vi "Working distances and rectangle.vi"() -> ()   [LabVIEW 2017]
uses:
  <vilib>/Simulation/Scripting/Companion Diagram/SimConfigNode/SimParams.ctl
  <vilib>/Simulation/Scripting/Companion Diagram/SimConfigNode/_simSolvers.ctl
  <vilib>/Simulation/Implementation/Shared/SIMSCR Execution Mode.ctl
  <vilib>/Simulation/Param Hierarchy/Typedefs/SIMPH Param Control Actions.ctl
  <vilib>/Simulation/Implementation/Shared/NILVSim_ParamChanged.vi
  <vilib>/Simulation/Implementation/Shared/NILVSIM_BeginStep.vi
  <vilib>/Simulation/Implementation/Shared/NILVSim_Manager.vi
  <vilib>/Utility/error.llb/Clear Errors.vi
  <vilib>/Simulation/Implementation/Shared/NILVSim_FinalizeModel.vi
  <vilib>/DAQmx/read.llb/DAQmx Read (Counter DBL 1Chan 1Samp).vi
  <vilib>/DAQmx/read.llb/DAQmx Read (Digital Bool 1Line 1Point).vi
  917b7e52-755f-4d44-bea8-9e7c9beac24e.vi
  a58f9967-76f1-4ebc-ad3d-26e75a3ca160.vi
  <vilib>/DAQmx/write.llb/DAQmx Write (Analog DBL 1Chan 1Samp).vi
  <vilib>/DAQmx/create/channels.llb/DAQmx Create Channel (AO-Voltage-Basic).vi
  <vilib>/DAQmx/create/channels.llb/DAQmx Create Channel (DI-Digital Input).vi
  <vilib>/DAQmx/create/channels.llb/DAQmx Create Channel (CI-Count Edges).vi
  <vilib>/Simulation/Implementation/Shared/SIM Unbundle Sim Info.vi
  <vilib>/Simulation/Implementation/Shared/NILVSim_Initialize.vi
  <vilib>/Simulation/Utility/Implementation/NILVSim Get Time and IsAcceptedStep.vi
  <vilib>/Simulation/Implementation/Shared/SIMSH Read Queue.vi
  <vilib>/Simulation/Implementation/Shared/NILVSim_GetModelError.vi
  <vilib>/Simulation/Implementation/Shared/SIM Bundle Sim Info.vi
  <vilib>/DAQmx/miscellaneous.llb/DAQmx Fill In Error Info.vi
  <vilib>/Simulation/Implementation/XNodeFramework/SimXNode/SimX.xnode
  <vilib>/Simulation/Model Libraries/PID/SIM PID (Parallel).vi
  <vilib>/Simulation/Model Libraries/PID/SIM PID.vi
  <vilib>/Simulation/Scripting/Companion Diagram/SimConfigNode/SimDog.xnode
  <vilib>/Simulation/Model Libraries/PID/SIM PID (Academic).vi
  <vilib>/Simulation/Implementation/Shared/NI_SIM_Implementation.lvlib
panel:
  out "circle reset":bool
  in  "part circle":enum16{"d", "c", "b", "a"}(ring)
  in  "Raduis":dbl
  out "at 2f":bool
  out "Step 2J":bool
  out "Step 2H":bool
  out "Shape drawing steps":enum16{"corner", "1st switch", "reverse"}(ring)
  out "Step 2D":bool
  out "Step 2C":bool
  out "c":bool
  in  "height":dbl
  in  "length":dbl
  in  "part":T1(ring)=enum."a"
  out "Step 2A":bool
  out "Step 2B":bool
  in  "Has encoders been reset?":enum16{"don't reset", "reset"}(ring)
  out "x distance currently being travelled":dbl
  out "y distance currently being travelled":dbl
  out "error calced":dbl
  out "p1 dis 2":dbl
  out "p1 dis":dbl
  out "error y":dbl
  out "calc distance y":dbl
  out "Boolean 2":bool
  out "calc distanc x":dbl
  out "error":dbl
  out "reached1":bool
  out "reached":bool
  out "Numeric":dbl
  in  "Draw rectangle":bool
  in  "Draw circle":bool
  out "In drawing mode":bool
  in  "Right-Down":bool
  in  "Left-Up":bool
  in  "Left-Down":bool
  in  "Right-Up":bool
  in  "right":bool
  in  "left":bool
  in  "motor 2":dbl(slide)=1.5 scale=-10.0..10.0
  in  "down":bool
  in  "up":bool
  in  "Y Length":dbl=30.0
  in  "X Length":dbl=30.0
  in  "Motor 2 encoder":tag="Dev1/ctr1"
  out "Pulses M2":dbl format="%.2f"
  in  "Motor 1 encoder":tag="Dev1/ctr0"
  out "Pulses M1":dbl format="%.2f"
  out "Right":bool
  out "Bottom":bool
  out "Left":bool
  out "Top":bool
  in  "Switch 4/Line 3":tag="Dev1/port0/line3"
  in  "Switch 3/Line 2":tag="Dev1/port0/line2"
  in  "Switch 2/Line 1":tag="Dev1/port0/line1"
  in  "Switch 1/Line 0":tag="Dev1/port0/line0"
  in  "Motor stop":bool
  in  "Motor 1":tag="Dev1/ao0"
  in  "max Voltage":dbl=10.0
  in  "Min Voltage":dbl=-10.0
  in  "Motor 2":tag="Dev1/ao1"
  in  "motor 1":dbl(slide)=1.5 scale=-10.0..10.0
  in  "stop":bool
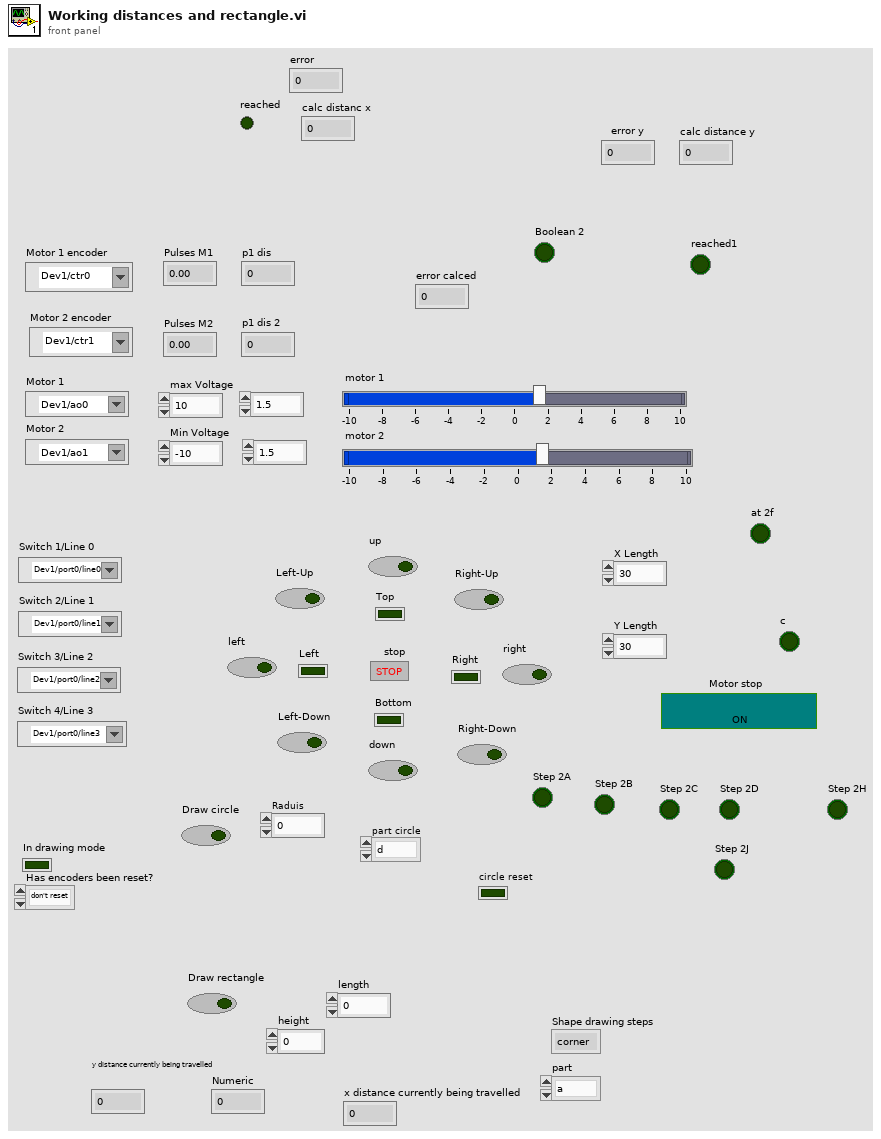
[diagram p1: front panel]
types:
  T1 = enum16{"nothing", "j", "i", "h", "g", "f", "e", "d", "c", "b", "a"}
  T2 = enum16{"Simulate to Completion", "Single Time-Step Simulation (Fixed Step Only)"}
  T3 = typedef "SIMSCR Execution Mode.ctl" = enum16{"Simulate to Completion", "Single Time-Step Simulation (Fixed Step Only)"}
  T4 = typedef "SIMPH Param Control Actions.ctl" = enum16{"get params", "set params"}
  T5 = cluster{"SIMSH Sim Time":dbl, "SIM PID Derivative Gain.vi":cluster{"output":dbl}, "SIM PID Derivative Gain.vi - SIMSH":cluster{"SIMSH Sim Time":dbl, "t 3":dbl, "Select 2":cluster{"s? t:f":dbl}, "Equal?":cluster{"x = y?":bool}, "Or":cluster{"x .or. y?":bool}, "Equal To 0?":cluster{"x = 0?":bool}}, "High Frequency [s] (Tf)":dbl, "Gain":cluster{"output":dbl}, "Summation":cluster{"Result":dbl}, "Integral Gain - series.vi":cluster{"output":dbl}, "Integral Gain - series.vi - SIMSH":cluster{"SIMSH Sim Time":dbl, "Select 2":cluster{"s? t:f":dbl}, "integral in gain?":bool, "Integrator":cluster{"output y(t)":dbl}, "Gain 2":cluster{"output":dbl}, "Select":cluster{"s? t:f":dbl}, "Equal To 0?":cluster{"x = 0?":bool}, "Reciprocal":cluster{"1/x":dbl}}}
  T6 = typedef "SimParams.ctl" = cluster{"Initial Time (s)":dbl, "Final Time (s)":dbl, "Step Size (s)":dbl, "ODE Solver":T7, "Minimum Step Size (s)":dbl, "Maximum Step Size (s)":dbl, "Relative Tolerance":dbl, "Absolute Tolerance":dbl, "Software Timing":bool, "Initial Step Size (s)":dbl, "Automatic Fixed Step Size?":bool, "Automatic Discrete Step Size?":bool, "Discrete Step Size (s)":dbl, "Calculate using Time Step":bool, "Solver Wired?":bool, "Prev.Frm.Expected End":u64, "Prev.Frm.Actual End":u64, "Prev.Frm.Finished Late?":bool, "Prev.Iter.Expected End":u64, "Prev.Iter.Actual End":u64, "Prev.Iter.Finished Late?":bool, "Expected Iteration Start":u64, "Actual Iteration Start":u64, "Expected Frame Start":u64, "Actual Frame Start":u64, "Source Name":string, "Name":string, "Period":i64, "Deadline":i64, "Offset":i64, "Start":i64, "Priority":i32, "Timeout":i32, "Processor":i32, "Mode":enum32{"No Change", "Process missed periods, maintain original phase", "Discard missed periods, maintain original phase", "Process missed periods, ignore original phase", "Discard missed periods, ignore original phase"}, "Wakeup reason":enum32{"Normal", "Aborted", "Asynchronous wakeup", "Timing source error", "Timed loop error", "Timeout"}, "Error":errorcluster, "Source Type":string, "Secondary Source Type":string, "Global End Time":u64, "Global Start Time":u64, "Full Solver Reset":bool, "Execution Mode":T3, "Nan/Inf Check":bool, "Custom Solver Library":string, "Solver Is Variable":bool, "custom solver name":string, "Signal Collection Decimation":u32}
  T7 = typedef "_simSolvers.ctl" = enum16{"Runge-Kutta 1 (Euler)", "Runge-Kutta 2", "Runge-Kutta 3", "Runge-Kutta 4", "Runge-Kutta 23 (variable)", "Runge-Kutta 45 (variable)", "BDF (variable)", "Adams-Moulton (variable)", "Rosenbrock (variable)", "Discrete States Only", "SDIRK 4 (variable)", "Radau 5 (variable)", "Radau 9 (variable)", "Radau 13 (variable)", "Radau [Variable Order] (variable)", "Gear's Method (variable)", "Linearizer", "State Query", "Trim Eval", "Custom Solver"}
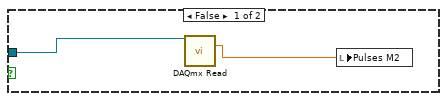
[diagram p2: hidden frame]
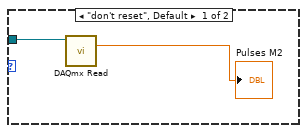
[diagram p3: hidden frame]
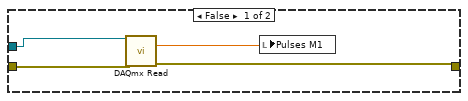
[diagram p4: hidden frame]
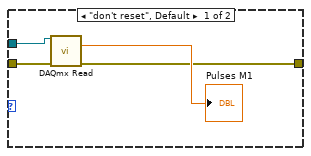
[diagram p5: hidden frame]
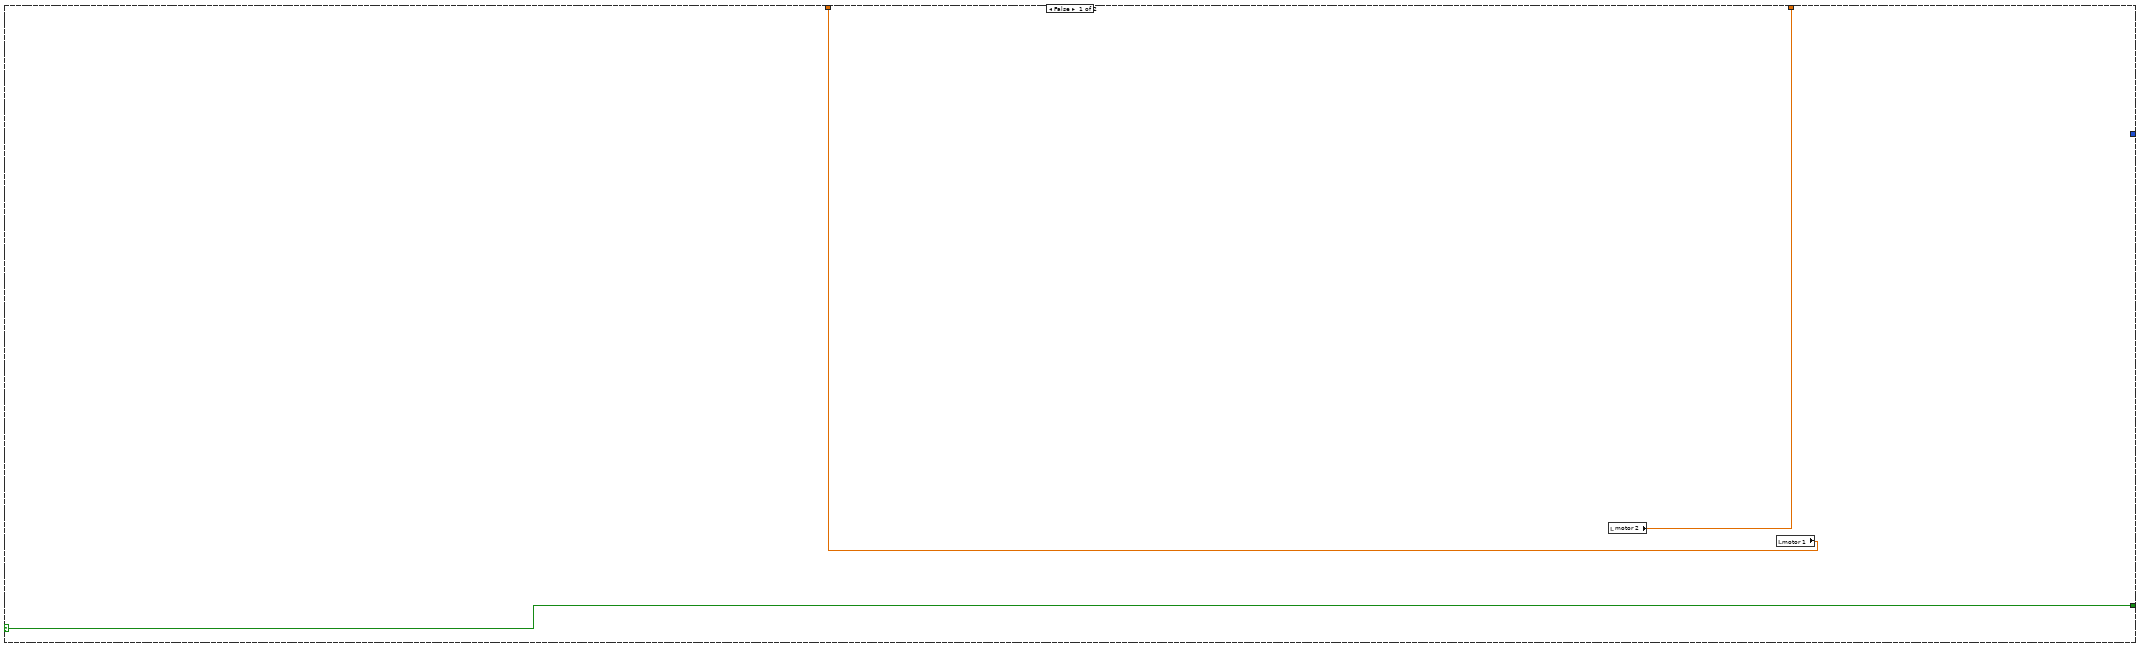
[diagram p6: hidden frame]
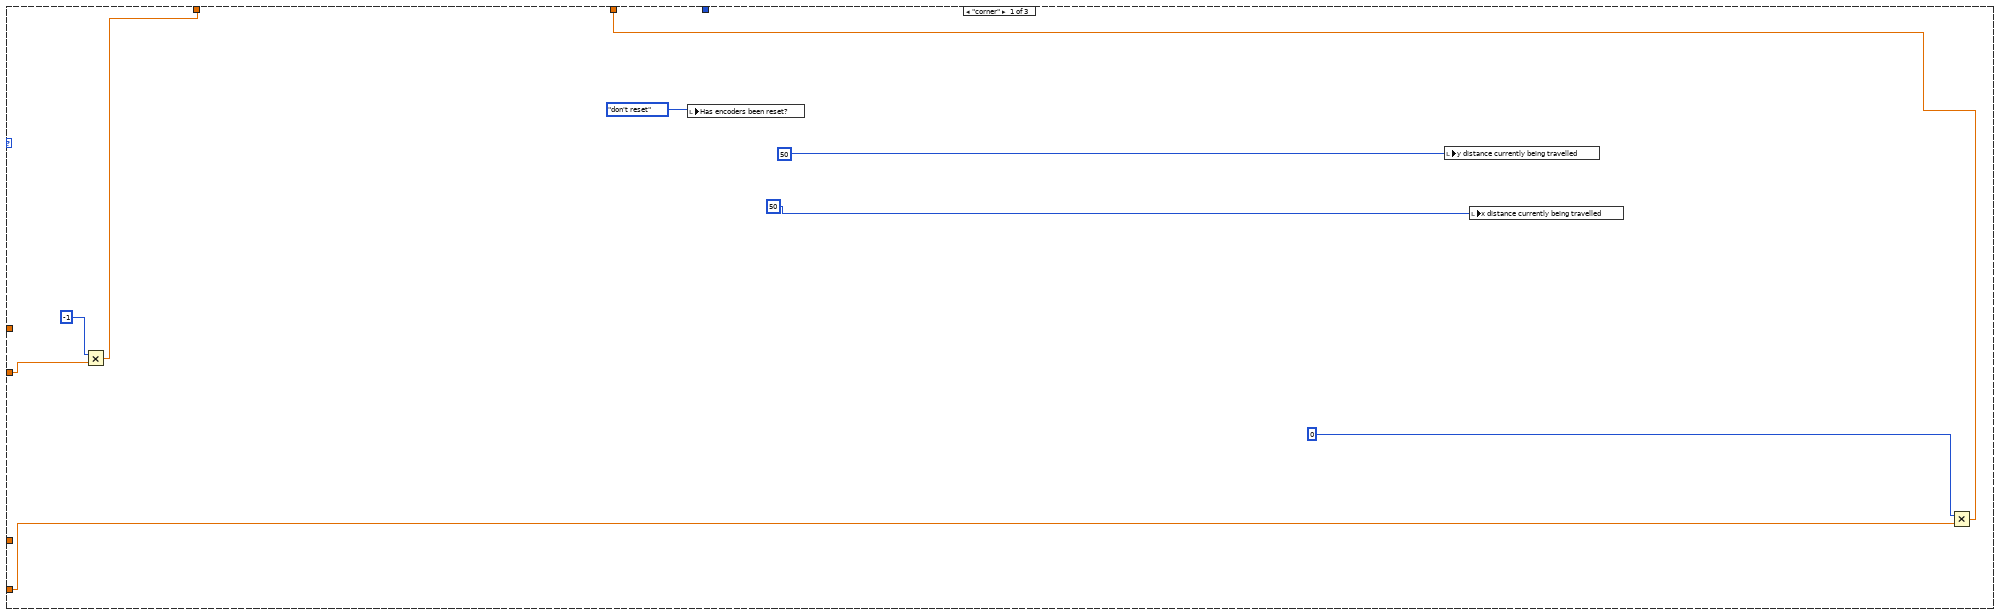
[diagram p7: hidden frame]
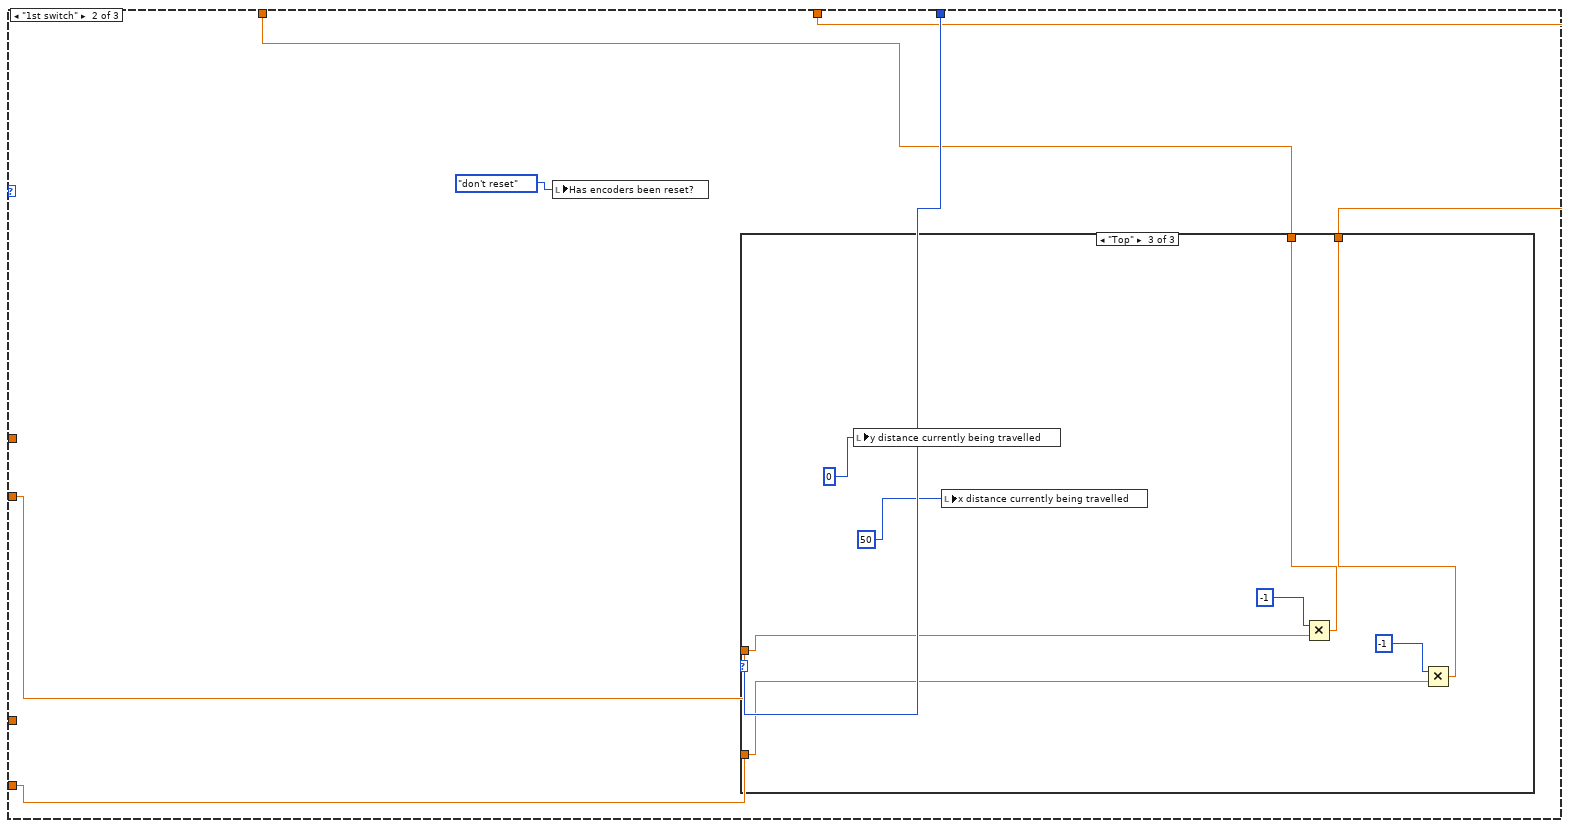
[diagram p8: hidden frame]
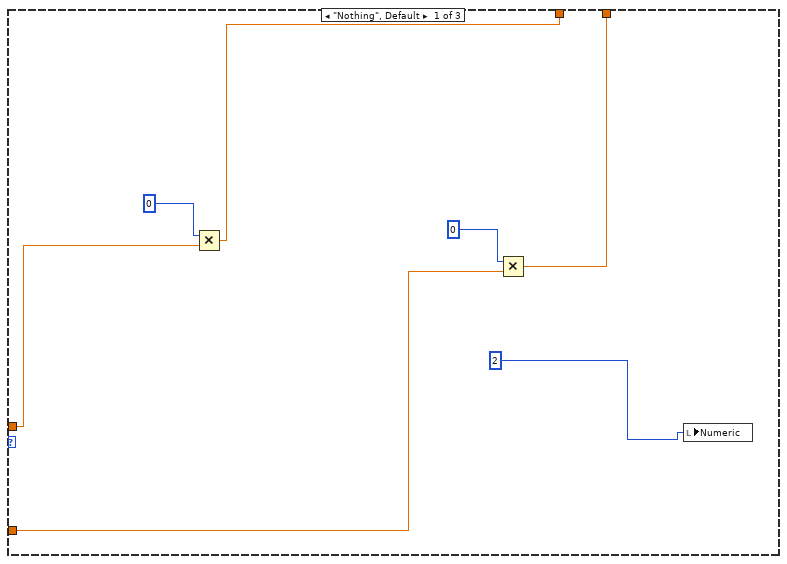
[diagram p9: hidden frame]
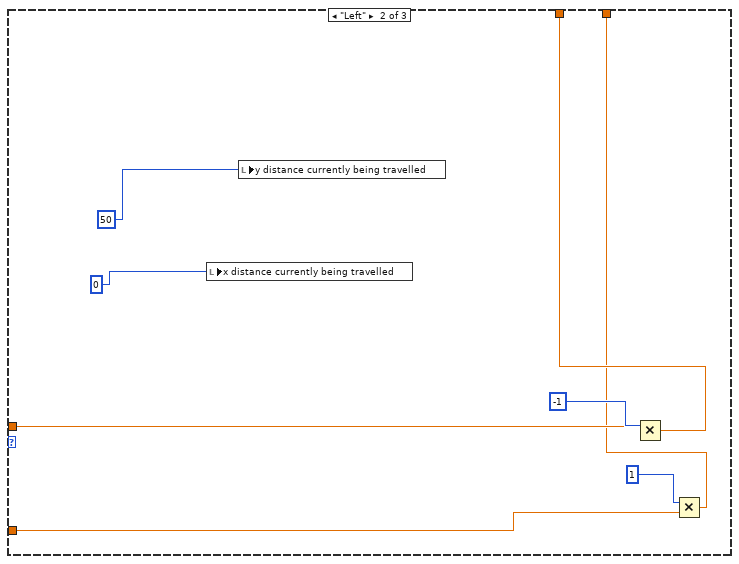
[diagram p10: hidden frame]
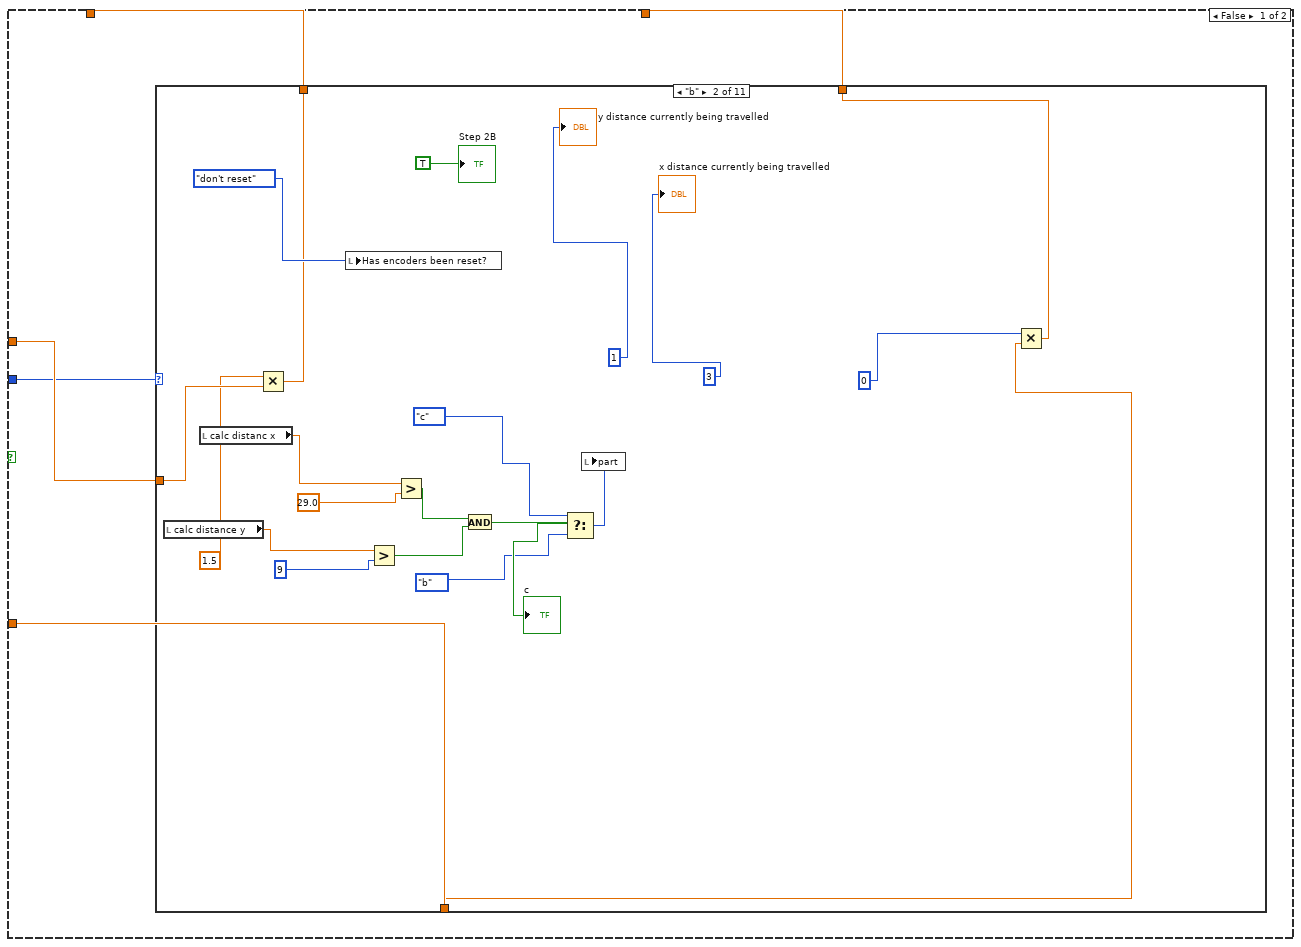
[diagram p11: hidden frame]
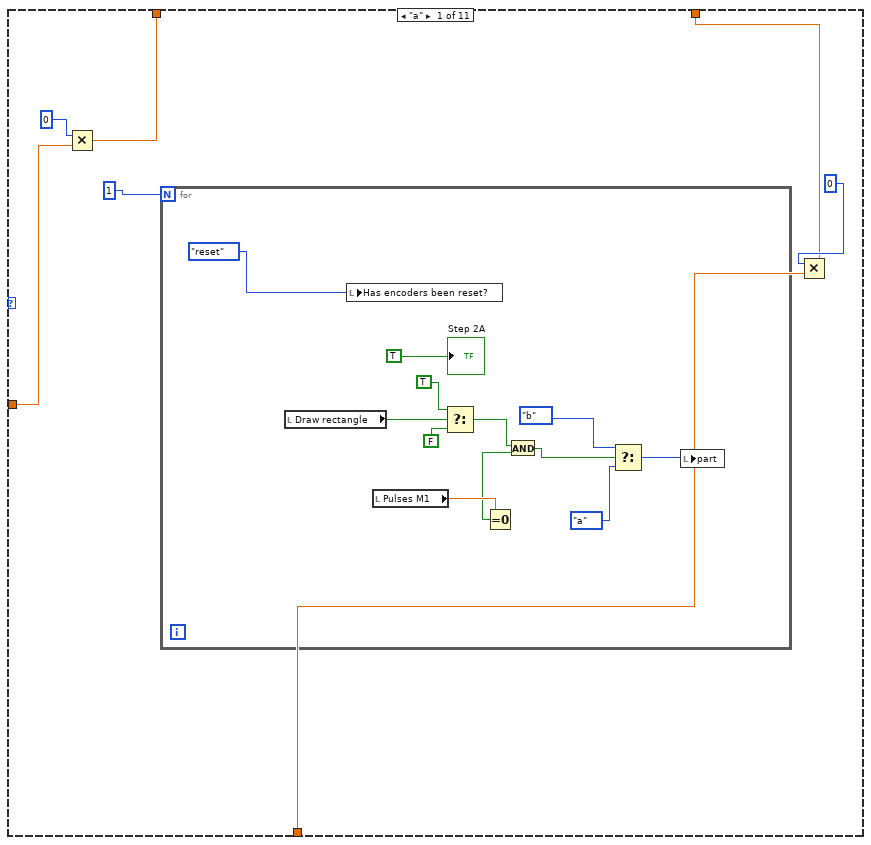
[diagram p12: hidden frame]
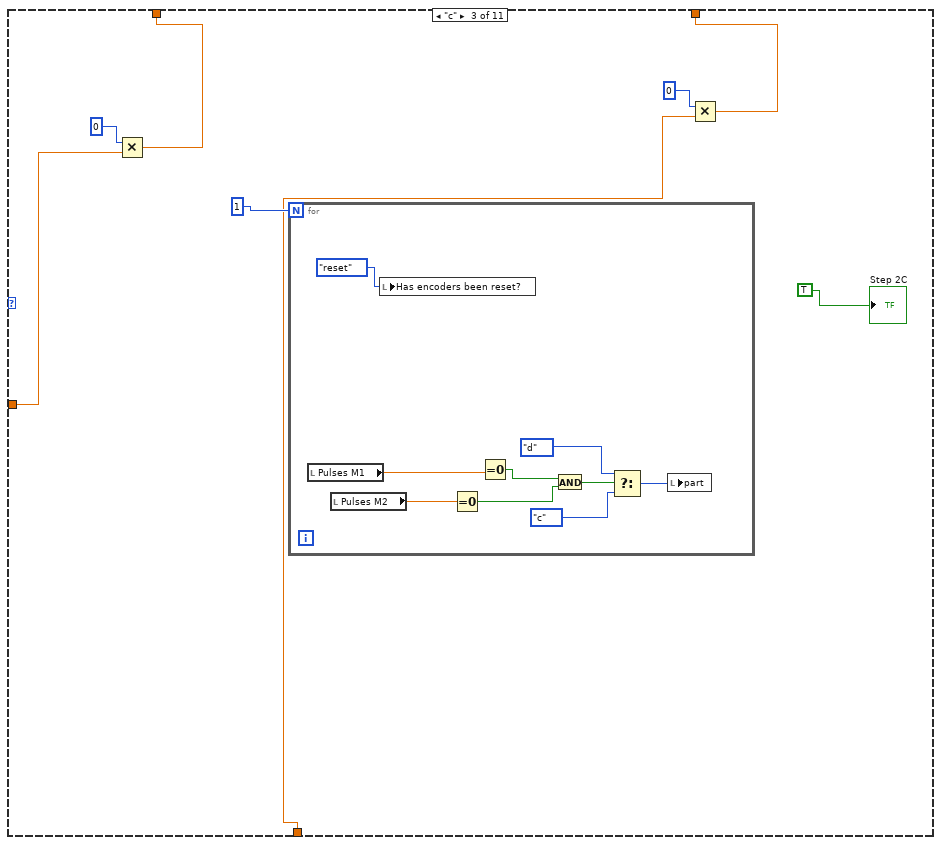
[diagram p13: hidden frame]
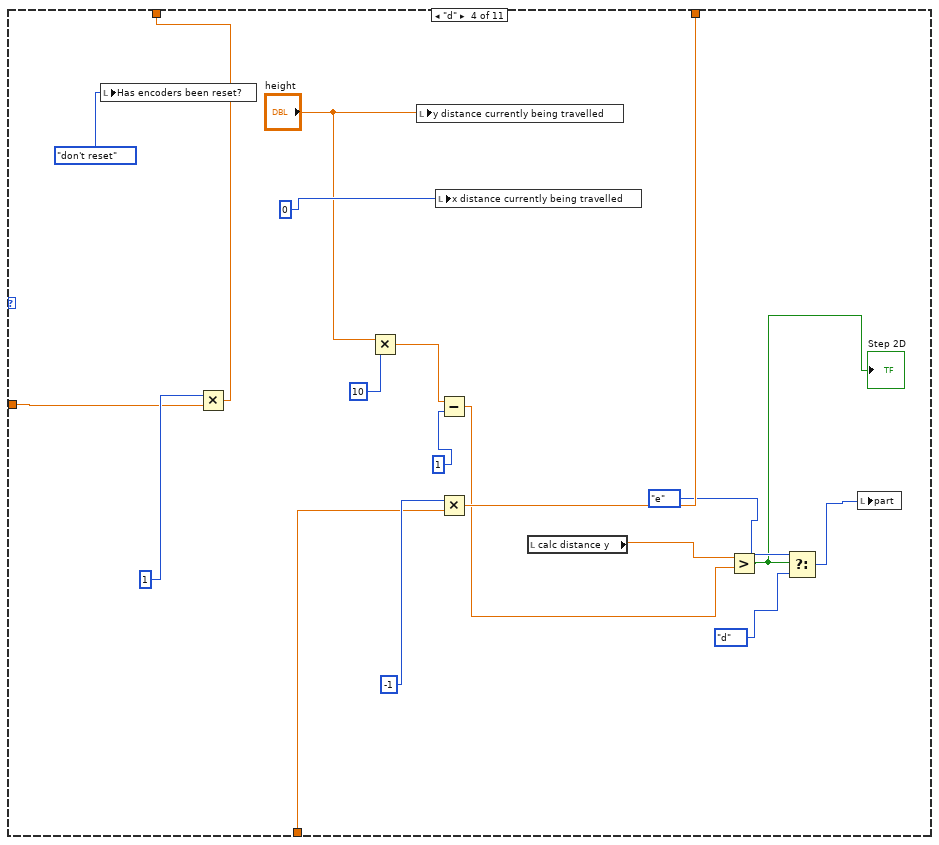
[diagram p14: hidden frame]
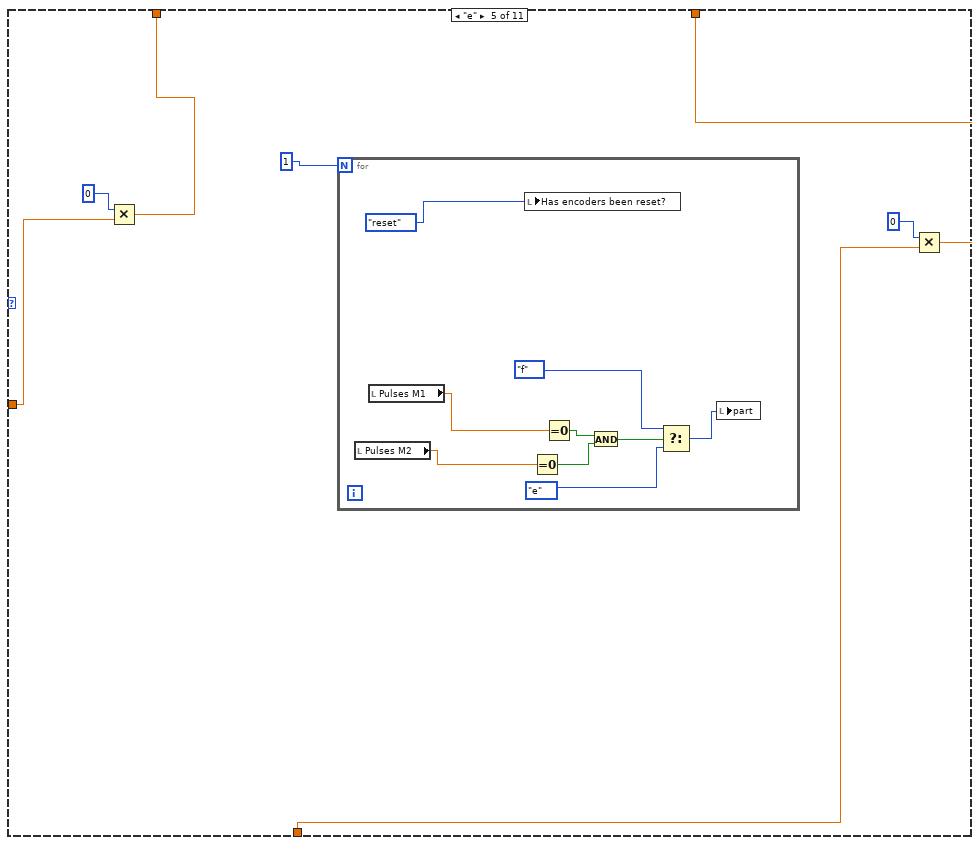
[diagram p15: hidden frame]
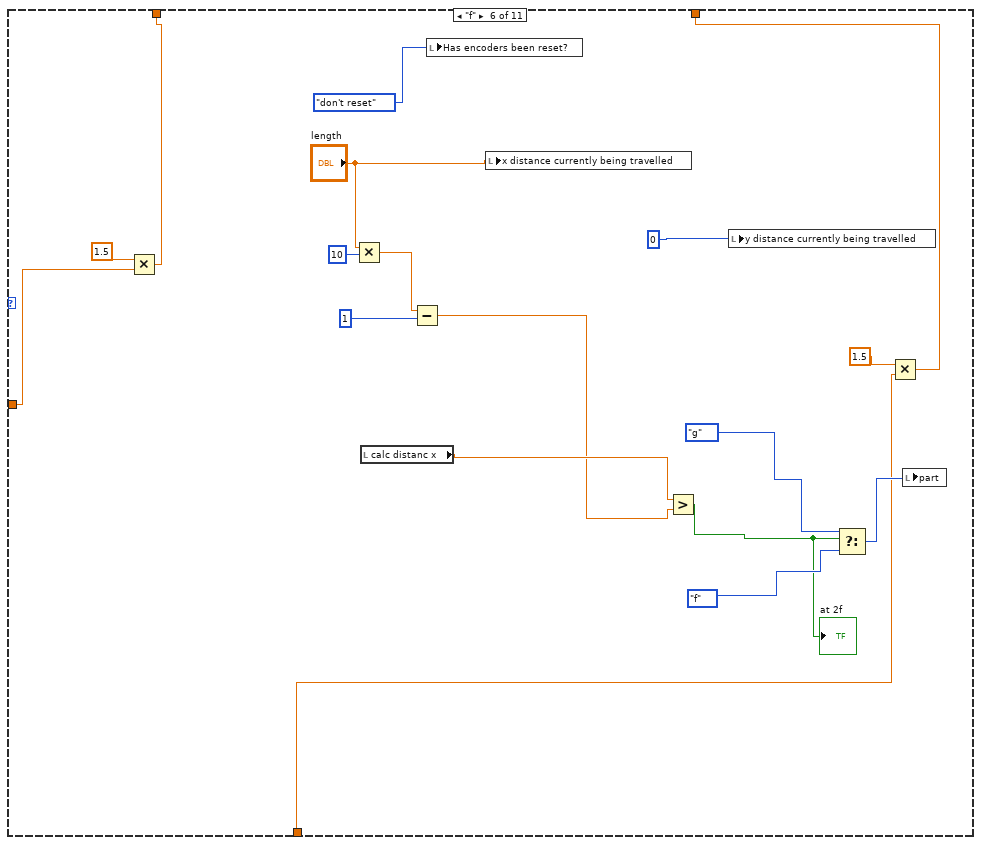
[diagram p16: hidden frame]
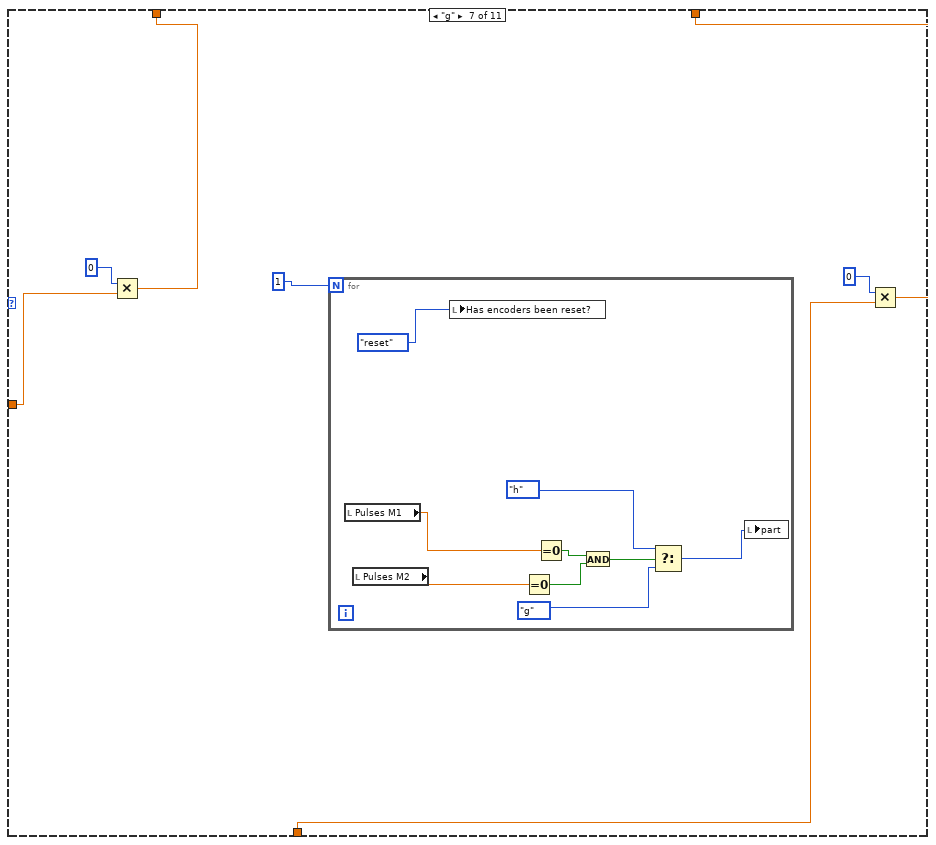
[diagram p17: hidden frame]
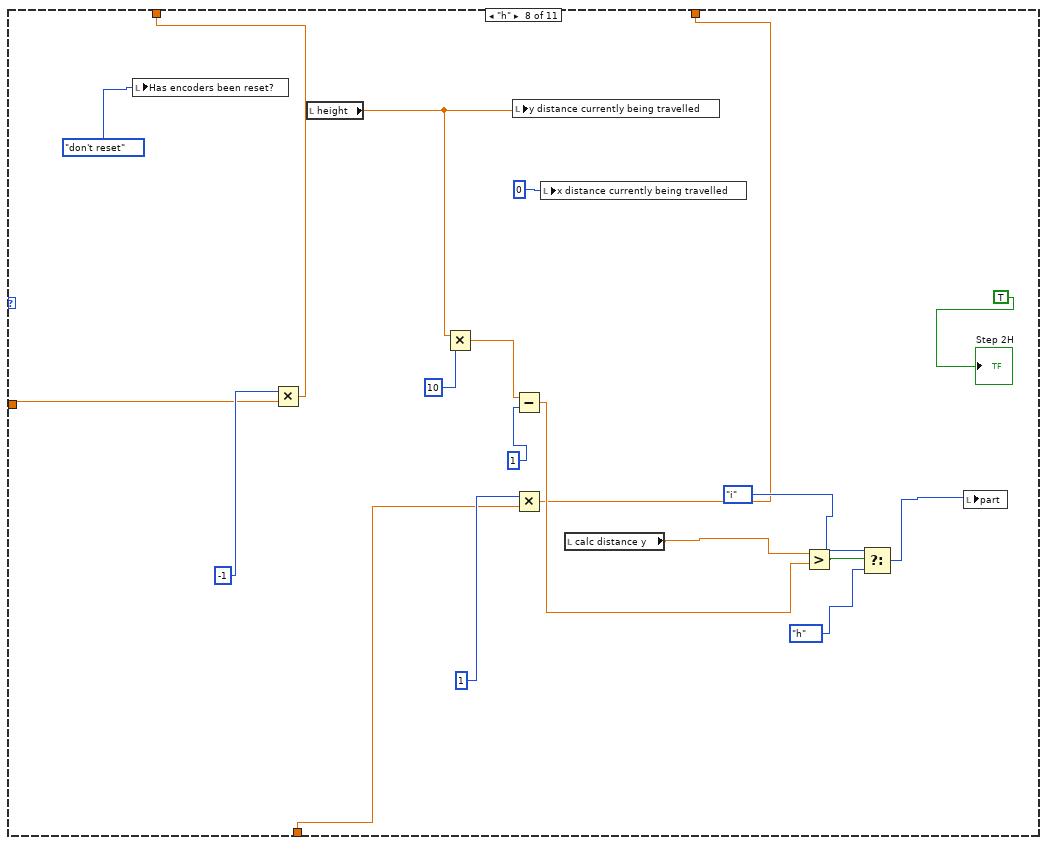
[diagram p18: hidden frame]
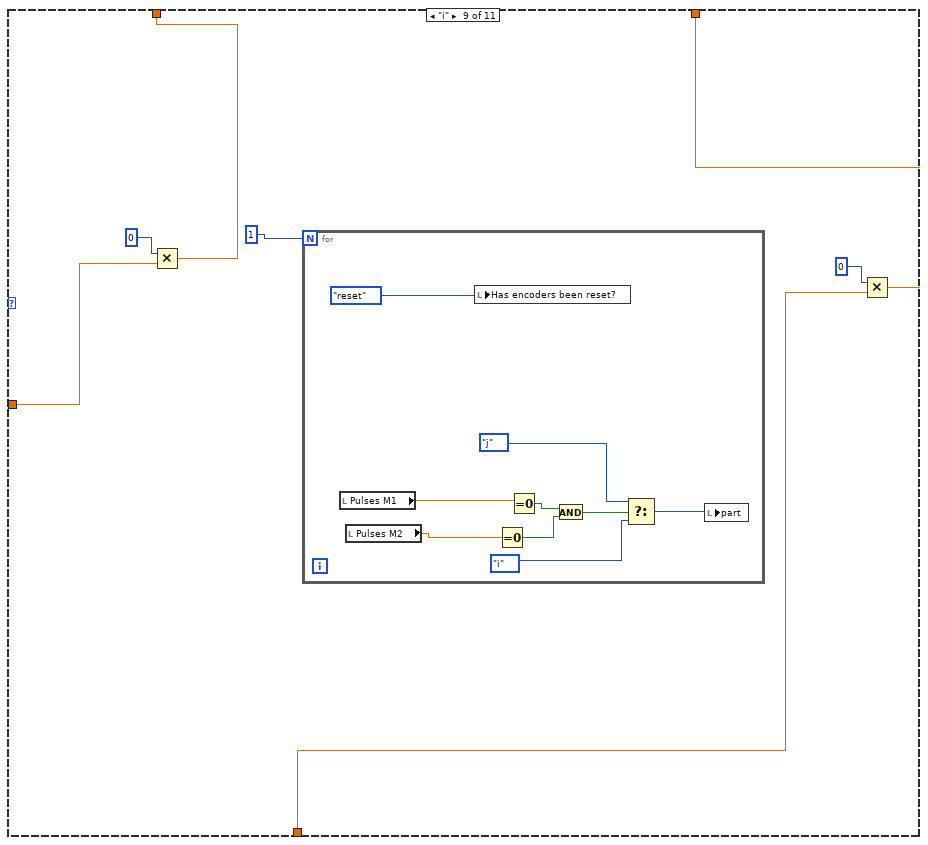
[diagram p19: hidden frame]
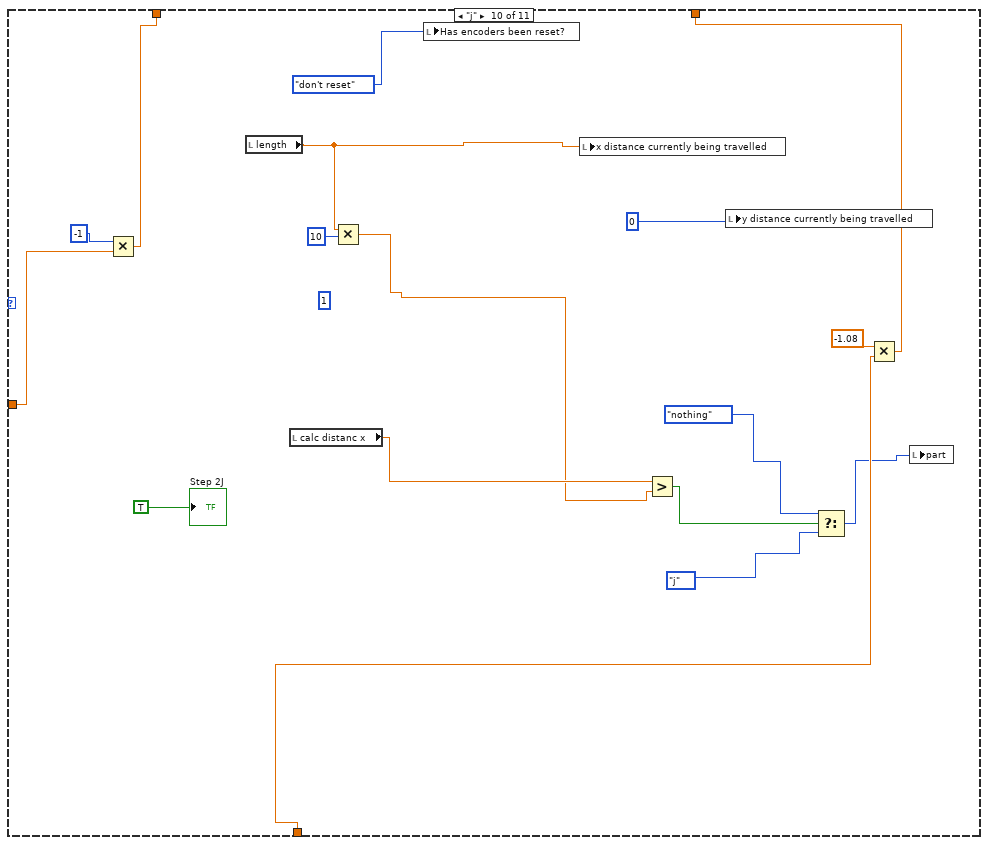
[diagram p20: hidden frame]
diagram:
  n1 = call-poly <vilib>:"DAQmx Create Virtual Channel.vi"("lines"="Switch 1/Line 0") -> ("task out"=w36:refnum<k21>, "error out"=w32:errorcluster)  [unwired: 13 in]
  n2 = call-poly <vilib>:"DAQmx Create Virtual Channel.vi"("lines"="Switch 2/Line 1") -> ("task out"=w35:refnum<k21>, "error out"=w31:errorcluster)  [unwired: 13 in]
  n3 = call-poly <vilib>:"DAQmx Create Virtual Channel.vi"("lines"="Switch 3/Line 2") -> ("task out"=w34:refnum<k21>, "error out"=w30:errorcluster)  [unwired: 13 in]
  n4 = call-poly <vilib>:"DAQmx Create Virtual Channel.vi"("lines"="Switch 4/Line 3") -> ("task out"=w33:refnum<k21>, "error out"=w29:errorcluster)  [unwired: 13 in]
  n5 = call <vilib>:"DAQmx Start Task.vi"("task/channels in"=w36, "error in"=w32) -> ("task out"=w28:refnum<k21>, "error out"=w26:errorcluster)  [unwired: 12 in]
  n6 = call <vilib>:"DAQmx Start Task.vi"("task/channels in"=w35, "error in"=w31) -> ("task out"=w24:refnum<k21>, "error out"=w21:errorcluster)  [unwired: 12 in]
  n7 = call <vilib>:"DAQmx Start Task.vi"("task/channels in"=w34, "error in"=w30) -> ("task out"=w23:refnum<k21>, "error out"=w20:errorcluster)  [unwired: 12 in]
  n8 = call <vilib>:"DAQmx Start Task.vi"("task/channels in"=w33, "error in"=w29) -> ("task out"=w22:refnum<k21>, "error out"=w19:errorcluster)  [unwired: 12 in]
  n9 = call-poly <vilib>:"DAQmx Create Virtual Channel.vi"("maximum value"="max Voltage", "minimum value"="Min Voltage", "physical channels"="Motor 1") -> ("task out"=w46:refnum<k21>, "error out"=w42:errorcluster)  [unwired: 11 in]
  n10 = call-poly <vilib>:"DAQmx Create Virtual Channel.vi"("counter"="Motor 2 encoder") -> ("task out"=w6:refnum<k21>)  [unwired: 13 in, 1 out]
  n11 = call-poly <vilib>:"DAQmx Create Virtual Channel.vi"("maximum value"="max Voltage", "minimum value"="Min Voltage", "physical channels"="Motor 2") -> ("task out"=w49:refnum<k21>, "error out"=w41:errorcluster)  [unwired: 11 in]
  n12 = call-poly <vilib>:"DAQmx Create Virtual Channel.vi"("counter"="Motor 1 encoder") -> ("task out"=w7:refnum<k21>, "error out"=w2:errorcluster)  [unwired: 13 in]
  n13 = call <vilib>:"DAQmx Start Task.vi"("task/channels in"=w6) -> ("task out"=w1:refnum<k21>)  [unwired: 13 in, 1 out]
  n14 = call <vilib>:"DAQmx Start Task.vi"("task/channels in"=w7) -> ("task out"=w3:refnum<k21>)  [unwired: 13 in, 1 out]
  n15 = while {
    tunnel: w49 -> [w203]
    tunnel: [w200] -> w48
    tunnel: w46 -> [w197]
    tunnel: [w196] -> w45
    tunnel: w42 -> [w194]
    tunnel: w41 -> [w193]
    tunnel: w28 -> [w187]
    tunnel: [w186] -> w27
    tunnel: w26 -> [w185]
    tunnel: [w184] -> w25
    tunnel: w24 -> [w183]
    tunnel: w23 -> [w182]
    tunnel: w22 -> [w181]
    tunnel: w21 -> [w180]
    tunnel: w20 -> [w179]
    tunnel: w19 -> [w178]
    tunnel: [w177] -> w18
    tunnel: [w176] -> w17
    tunnel: [w175] -> w16
    tunnel: [w174] -> w15
    tunnel: [w173] -> w14
    tunnel: [w172] -> w13
    tunnel: [w69] -> w10
    tunnel: w3 -> [w71]
    tunnel: w2 -> [w70]
    tunnel: w1 -> [w67]
    stop <- "stop" stop-if-true
    n16 = Or(x="Draw circle", y="Draw rectangle") -> (x .or. y?=w101:bool)
    n17 = local read "y distance currently being travelled"() -> (w73:dbl)
    n18 = Select(t=1, s="up", f=0) -> (s? t:f=w148:i32)
    n19 = Select(t=10, s="left", f=0) -> (s? t:f=w146:i32)
    n20 = Select(t=2, s="down", f=0) -> (s? t:f=w147:i32)
    n21 = Select(t=100, s="Right-Up", f=0) -> (s? t:f=w144:i32)
    n22 = Select(t=200, s="Left-Down", f=0) -> (s? t:f=w143:i32)
    n23 = Select(t=20, s="right", f=0) -> (s? t:f=w145:i32)
    n24 = Select(t=1000, s="Left-Up", f=0) -> (s? t:f=w142:i32)
    n25 = Select(t=2000, s="Right-Down", f=0) -> (s? t:f=w128:i32)
    n26 = Add(x=w148, y=w147) -> (x+y=w141:i32)
    n27 = Add(x=w146, y=w145) -> (x+y=w140:i32)
    n28 = Add(x=w144, y=w143) -> (x+y=w139:i32)
    n29 = Add(x=w142, y=w128) -> (x+y=w127:i32)
    n30 = local read "Draw rectangle"() -> (w81:bool)
    n31 = local read "Draw circle"() -> (w82:bool)
    n32 = Add(x=w141, y=w140) -> (x+y=w138:i32)
    n33 = Add(x=w139, y=w127) -> (x+y=w126:i32)
    n34 = Or(x=w82, y=w81) -> (x .or. y?=w80:bool)
    n35 = call-poly <vilib>:"DAQmx Read.vi"("task/channels in"=w187, "error in"=w185) -> ("task out"=w186:refnum<k21>, "data"=w103:bool, "error out"=w184:errorcluster)  [unwired: 11 in]
    "Top" <- w103
    n36 = call-poly <vilib>:"DAQmx Read.vi"("task/channels in"=w183, "error in"=w180) -> ("task out"=w177:refnum<k21>, "data"=w112:bool, "error out"=w174:errorcluster)  [unwired: 11 in]
    "Bottom" <- w112
    n37 = call-poly <vilib>:"DAQmx Read.vi"("task/channels in"=w182, "error in"=w179) -> ("task out"=w176:refnum<k21>, "data"=w111:bool, "error out"=w173:errorcluster)  [unwired: 11 in]
    "Right" <- w111
    n38 = call-poly <vilib>:"DAQmx Read.vi"("task/channels in"=w181, "error in"=w178) -> ("task out"=w175:refnum<k21>, "data"=w110:bool, "error out"=w172:errorcluster)  [unwired: 11 in]
    "Left" <- w110
    n39 = Select(t=w73, s=w80, f="Y Length") -> (s? t:f=w78:dbl)
    n40 = local read "Pulses M1"() -> (w68:dbl)
    n41 = Add(x=w138, y=w126) -> (x+y=w125:i32)
    n42 = Multiply(x=w78, y=10) -> (x*y=w51:dbl)
    n43 = local read "Pulses M2"() -> (w83:dbl)
    n44 = Divide(x=w83, y=52.56) -> (x/y=→"p1 dis 2":dbl)
    n45 = Divide(x=w68, y=52.56) -> (x/y=→"p1 dis":dbl)
    n46 = formula code="X=((PulseM1/52.56)+(PulseM2/52.56))/2.0;\nY=((PulseM1/52.56)-(-PulseM2/52.56))/2.0;"("PulseM1"=w68, "PulseM2"=w83) -> ("X"=w54:dbl, "Y"=w52:dbl)
    "calc distanc x" <- w54
    "calc distance y" <- w52
    n47 = Subtract(x=w52, y=w51) -> (x-y=w53:dbl)
    "error y" <- w53
    n48 = local read "x distance currently being travelled"() -> (w72:dbl)
    n49 = local read "Draw rectangle"() -> (w75:bool)
    n50 = local read "Draw circle"() -> (w74:bool)
    n51 = Or(x=w75, y=w74) -> (x .or. y?=w63:bool)
    n52 = xnode "PID"("Error"=w53) -> ("Output"=w90:dbl)  [unwired: 2 in, 11 out]
    n53 = Select(t=w72, s=w63, f="X Length") -> (s? t:f=w76:dbl)
    n54 = Multiply(x=w76, y=10) -> (x*y=w55:dbl)
    n55 = Subtract(x=w54, y=w55) -> (x-y=w56:dbl)
    "error calced" <- w56
    n56 = case shown="20" w125 {
      tunnel: "motor 1" -> [w1034 w1037 w1040 w1047 w1051 w1055 w1061 w1067 w1073 w1078 w1085]
      tunnel: "motor 2" -> [w1031 w1039 w1042 w1045 w1050 w1053 w1059 w1065 w1071 w1079 w1084]
      tunnel: [w1030 w1039 w1041 w1044 w1050 w1052 w1058 w1064 w1070 w1076 w1083] -> w119
      tunnel: [w1033 w1036 w1040 w1046 w1051 w1054 w1060 w1066 w1072 w1077 w1082] -> w121
      frame 0, Default {
        n57 = Multiply(x=0, y=w1034) -> (x*y=w1033:dbl)
        n58 = Multiply(x=0, y=w1031) -> (x*y=w1030:dbl)
      }
      frame 1 {
        n59 = Multiply(x=-1, y=w1037) -> (x*y=w1036:dbl)
      }
      frame 2 {
        n60 = Multiply(x=-1.003, y=w1042) -> (x*y=w1041:dbl)
      }
      frame 10 {
        n61 = Multiply(x=-1, y=w1047) -> (x*y=w1046:dbl)
        n62 = Multiply(x=-1.1, y=w1045) -> (x*y=w1044:dbl)
      }
      frame 20 {
      }
      frame 100 {
        n63 = Multiply(x=0, y=w1055) -> (x*y=w1054:dbl)
        n64 = Multiply(x=1, y=w1053) -> (x*y=w1052:dbl)
      }
      frame 200 {
        n65 = Multiply(x=0, y=w1061) -> (x*y=w1060:dbl)
        n66 = Multiply(x=-1, y=w1059) -> (x*y=w1058:dbl)
      }
      frame 1000 {
        n67 = Multiply(x=-1, y=w1067) -> (x*y=w1066:dbl)
        n68 = Multiply(x=0, y=w1065) -> (x*y=w1064:dbl)
      }
      frame 2000 {
        n69 = Multiply(x=1, y=w1073) -> (x*y=w1072:dbl)
        n70 = Multiply(x=0, y=w1071) -> (x*y=w1070:dbl)
      }
      frame 4000 {
        n71 = Multiply(x=-1, y=w1078) -> (x*y=w1077:dbl)
        n72 = Multiply(x=0, y=w1079) -> (x*y=w1076:dbl)
      }
      frame 8000 {
        n73 = Multiply(x=-1, y=w1085) -> (x*y=w1082:dbl)
        n74 = Multiply(x=0, y=w1084) -> (x*y=w1083:dbl)
      }
    }
    n75 = Less?(x=0.5, y=w90) -> (x < y?=w88:bool)
    n76 = Less?(x=-0.5, y=w90) -> (x < y?=w89:bool)
    n77 = xnode "PID 2"("Error"=w56) -> ("Output"=w93:dbl)  [unwired: 2 in, 11 out]
    "error" <- w93
    n78 = local read "Numeric"() -> (w60:dbl)
    n79 = Or(x=w88, y=w89) -> (x .or. y?=w96:bool)
    "reached1" <- w96
    n80 = Or(x=w112, y=w111) -> (x .or. y?=w170:bool)
    n81 = local read "Draw circle"() -> (w65:bool)
    n82 = local read "Draw rectangle"() -> (w64:bool)
    n83 = And(x=w110, y=w103) -> (x .and. y?=w61:bool)
    n84 = Exclusive Or(1:w103, 2:w110) -> (0:w117:bool)
    n85 = Less?(x=0.5, y=w93) -> (x < y?=w95:bool)
    n86 = Select(t=1, s=w110, f=0) -> (s? t:f=w102:i32)
    n87 = Select(t=2, s=w103, f=w102) -> (s? t:f=w107:i32)
    n88 = Less?(x=-0.5, y=w93) -> (x < y?=w92:bool)
    n89 = Or(x=w95, y=w92) -> (x .or. y?=w97:bool)
    "reached" <- w97
    n90 = Select(t=1, s=w117, f=w60) -> (s? t:f=w116:dbl)
    n91 = Select(t=2, s=w61, f=w116) -> (s? t:f=w114:dbl)
    n92 = Or(x=w65, y=w64) -> (x .or. y?=w66:bool)
    n93 = call "Number To Enum.vim"("number"=w107, "enum type"=enum16{"Nothing", "Left", "Top"}."Nothing") -> ("number as enum"=w104:enum16{"Nothing", "Left", "Top"})
    n94 = case shown="True" w101 {
      selector: w101 -> [w731 w739]
      tunnel: [w731 w739] -> w124
      tunnel: [w730 w741] -> w123
      tunnel: [w729 w740] -> w122
      tunnel: w104 -> [_ w732]
      frame False {
        n95 = local read "motor 2"() -> (w729:dbl)
        n96 = local read "motor 1"() -> (w730:dbl)
      }
      frame True {
        n97 = local read "Numeric"() -> (w737:dbl)
        n98 = local read "Shape drawing steps"() -> (w734:enum16{"corner", "1st switch", "reverse"})
        n99 = Equal?(x=w737, y=2) -> (x = y?=w736:bool)
        n100 = Select(t=enum16{"corner", "1st switch", "reverse"}."reverse", s=w736, f=w734) -> (s? t:f=w733:enum16{"corner", "1st switch", "reverse"})
        n101 = local read "motor 2"() -> (w742:dbl)
        n102 = local read "motor 1"() -> (w743:dbl)
        n103 = case shown="\"reverse\"" w733 {
          tunnel: w732 -> [_ w758 _]
          tunnel: w743 -> [w750 w757 _]
          tunnel: w742 -> [w749 w756 _]
          tunnel: w743 -> [_ _ w788]
          tunnel: w742 -> [_ _ w787]
          tunnel: [w746 w755 w786] -> w741
          tunnel: [w745 w754 w785] -> w740
          frame "corner" {
            n104 = Multiply(x=-1, y=w750) -> (x*y=w746:dbl)
            n105 = local write "Has encoders been reset?"(enum16{"don't reset", "reset"}."don't reset") -> ()
            n106 = local write "y distance currently being travelled"(50) -> ()
            n107 = local write "x distance currently being travelled"(50) -> ()
            n108 = Multiply(x=0, y=w749) -> (x*y=w745:dbl)
          }
          frame "1st switch" {
            n109 = local write "Has encoders been reset?"(enum16{"don't reset", "reset"}."don't reset") -> ()
            n110 = case shown="\"Top\"" w758 {
              tunnel: [w763 w770 w779] -> w755
              tunnel: w757 -> [w765 w771 w777]
              tunnel: [w760 w768 w778] -> w754
              tunnel: w756 -> [w761 w769 w776]
              frame "Nothing", Default {
                n111 = Multiply(x=0, y=w765) -> (x*y=w763:dbl)
                n112 = Multiply(x=0, y=w761) -> (x*y=w760:dbl)
                n113 = local write "Numeric"(2) -> ()
              }
              frame "Left" {
                n114 = local write "x distance currently being travelled"(0) -> ()
                n115 = local write "y distance currently being travelled"(50) -> ()
                n116 = Multiply(x=-1, y=w771) -> (x*y=w770:dbl)
                n117 = Multiply(x=1, y=w769) -> (x*y=w768:dbl)
              }
              frame "Top" {
                n118 = local write "y distance currently being travelled"(0) -> ()
                n119 = local write "x distance currently being travelled"(50) -> ()
                n120 = Multiply(x=-1, y=w777) -> (x*y=w779:dbl)
                n121 = Multiply(x=-1, y=w776) -> (x*y=w778:dbl)
              }
            }
          }
          frame "reverse" {
            n122 = local read "Draw circle"() -> (w782:bool)
            n123 = case shown="True" w782 {
              tunnel: w788 -> [w793 w978]
              tunnel: w787 -> [w792 w977]
              tunnel: [w791 w978] -> w786
              tunnel: [w790 w977] -> w785
              tunnel: "part" -> [w789 _]
              frame False {
                n124 = case shown="\"b\"" w789 {
                  tunnel: w793 -> [w799 w829 w837 w865 w872 w889 w905 w926 w940 w963 w974]
                  tunnel: w792 -> [w796 w826 w835 w862 w868 w886 w902 w921 w937 w961 w972]
                  tunnel: [w797 w828 w836 w863 w871 w888 w906 w925 w941 w962 w973] -> w791
                  tunnel: [w794 w825 w834 w861 w869 w885 w903 w920 w938 w960 w970] -> w790
                  frame "a" {
                    n125 = Multiply(x=0, y=w799) -> (x*y=w797:dbl)
                    n126 = for {
                      N: 1 -> [_]
                      n127 = local read "Draw rectangle"() -> (w801:bool)
                      n128 = local write "Has encoders been reset?"(enum16{"don't reset", "reset"}."reset") -> ()
                      n129 = local read "Pulses M1"() -> (w810:dbl)
                      n130 = Select(t=TRUE, s=w801, f=FALSE) -> (s? t:f=w804:bool)
                      n131 = Equal To 0?(x=w810) -> (x = 0?=w803:bool)
                      n132 = And(x=w804, y=w803) -> (x .and. y?=w802:bool)
                      n133 = Select(t=T1."b", s=w802, f=T1."a") -> (s? t:f=w809:T1)
                      n134 = local write "part"(w809) -> ()
                      "Step 2A" <- TRUE
                    }
                    n135 = Multiply(x=0, y=w796) -> (x*y=w794:dbl)
                  }
                  frame "b" {
                    n136 = local read "calc distance y"() -> (w813:dbl)
                    n137 = local read "calc distanc x"() -> (w814:dbl)
                    n138 = Multiply(x=1.5, y=w829) -> (x*y=w828:dbl)
                    n139 = local write "Has encoders been reset?"(enum16{"don't reset", "reset"}."don't reset") -> ()
                    n140 = Greater?(x=w813, y=9) -> (0:w819:bool)
                    n141 = Greater?(x=w814, y=29.0) -> (0:w818:bool)
                    n142 = And(x=w818, y=w819) -> (x .and. y?=w817:bool)
                    "c" <- w817
                    n143 = Select(t=T1."c", s=w817, f=T1."b") -> (s? t:f=w822:T1)
                    n144 = local write "part"(w822) -> ()
                    n145 = Multiply(x=0, y=w826) -> (x*y=w825:dbl)
                    "x distance currently being travelled" <- 3
                    "y distance currently being travelled" <- 1
                    "Step 2B" <- TRUE
                  }
                  frame "c" {
                    n146 = Multiply(x=0, y=w837) -> (x*y=w836:dbl)
                    n147 = for {
                      N: 1 -> [_]
                      n148 = local read "Pulses M1"() -> (w848:dbl)
                      n149 = local read "Pulses M2"() -> (w844:dbl)
                      n150 = local write "Has encoders been reset?"(enum16{"don't reset", "reset"}."reset") -> ()
                      n151 = Equal To 0?(x=w844) -> (x = 0?=w842:bool)
                      n152 = Equal To 0?(x=w848) -> (x = 0?=w843:bool)
                      n153 = And(x=w843, y=w842) -> (x .and. y?=w841:bool)
                      n154 = Select(t=T1."d", s=w841, f=T1."c") -> (s? t:f=w847:T1)
                      n155 = local write "part"(w847) -> ()
                    }
                    n156 = Multiply(x=0, y=w835) -> (x*y=w834:dbl)
                    "Step 2C" <- TRUE
                  }
                  frame "d" {
                    n157 = local write "Has encoders been reset?"(enum16{"don't reset", "reset"}."don't reset") -> ()
                    n158 = Multiply(x=1, y=w865) -> (x*y=w863:dbl)
                    n159 = Multiply(x="height", y=10) -> (x*y=w857:dbl)
                    n160 = local write "y distance currently being travelled"("height") -> ()
                    n161 = local write "x distance currently being travelled"(0) -> ()
                    n162 = Subtract(x=w857, y=1) -> (x-y=w854:dbl)
                    n163 = Multiply(x=-1, y=w862) -> (x*y=w861:dbl)
                    n164 = local read "calc distance y"() -> (w859:dbl)
                    n165 = Greater?(x=w859, y=w854) -> (0:w850:bool)
                    "Step 2D" <- w850
                    n166 = Select(t=T1."e", s=w850, f=T1."d") -> (s? t:f=w860:T1)
                    n167 = local write "part"(w860) -> ()
                  }
                  frame "e" {
                    n168 = Multiply(x=0, y=w872) -> (x*y=w871:dbl)
                    n169 = for {
                      N: 1 -> [_]
                      n170 = local read "Pulses M2"() -> (w876:dbl)
                      n171 = local read "Pulses M1"() -> (w877:dbl)
                      n172 = local write "Has encoders been reset?"(enum16{"don't reset", "reset"}."reset") -> ()
                      n173 = Equal To 0?(x=w876) -> (x = 0?=w882:bool)
                      n174 = Equal To 0?(x=w877) -> (x = 0?=w883:bool)
                      n175 = And(x=w883, y=w882) -> (x .and. y?=w881:bool)
                      n176 = Select(t=T1."f", s=w881, f=T1."e") -> (s? t:f=w875:T1)
                      n177 = local write "part"(w875) -> ()
                    }
                    n178 = Multiply(x=0, y=w868) -> (x*y=w869:dbl)
                  }
                  frame "f" {
                    n179 = Multiply(x=1.5, y=w889) -> (x*y=w888:dbl)
                    n180 = Multiply(x="length", y=10) -> (x*y=w896:dbl)
                    n181 = local read "calc distanc x"() -> (w899:dbl)
                    n182 = Subtract(x=w896, y=1) -> (x-y=w893:dbl)
                    n183 = local write "Has encoders been reset?"(enum16{"don't reset", "reset"}."don't reset") -> ()
                    n184 = local write "x distance currently being travelled"("length") -> ()
                    n185 = Greater?(x=w899, y=w893) -> (0:w884:bool)
                    "at 2f" <- w884
                    n186 = local write "y distance currently being travelled"(0) -> ()
                    n187 = Select(t=T1."g", s=w884, f=T1."f") -> (s? t:f=w898:T1)
                    n188 = Multiply(x=1.5, y=w886) -> (x*y=w885:dbl)
                    n189 = local write "part"(w898) -> ()
                  }
                  frame "g" {
                    n190 = Multiply(x=0, y=w905) -> (x*y=w906:dbl)
                    n191 = for {
                      N: 1 -> [_]
                      n192 = local read "Pulses M1"() -> (w910:dbl)
                      n193 = local read "Pulses M2"() -> (w909:dbl)
                      n194 = local write "Has encoders been reset?"(enum16{"don't reset", "reset"}."reset") -> ()
                      n195 = Equal To 0?(x=w909) -> (x = 0?=w916:bool)
                      n196 = Equal To 0?(x=w910) -> (x = 0?=w917:bool)
                      n197 = And(x=w917, y=w916) -> (x .and. y?=w915:bool)
                      n198 = Select(t=T1."h", s=w915, f=T1."g") -> (s? t:f=w912:T1)
                      n199 = local write "part"(w912) -> ()
                    }
                    n200 = Multiply(x=0, y=w902) -> (x*y=w903:dbl)
                  }
                  frame "h" {
                    n201 = local write "Has encoders been reset?"(enum16{"don't reset", "reset"}."don't reset") -> ()
                    n202 = Multiply(x=-1, y=w926) -> (x*y=w925:dbl)
                    n203 = local read "height"() -> (w923:dbl)
                    n204 = Multiply(x=w923, y=10) -> (x*y=w933:dbl)
                    n205 = local write "y distance currently being travelled"(w923) -> ()
                    n206 = Subtract(x=w933, y=1) -> (x-y=w930:dbl)
                    n207 = Multiply(x=1, y=w921) -> (x*y=w920:dbl)
                    n208 = local write "x distance currently being travelled"(0) -> ()
                    n209 = local read "calc distance y"() -> (w919:dbl)
                    n210 = Greater?(x=w919, y=w930) -> (0:w934:bool)
                    n211 = Select(t=T1."i", s=w934, f=T1."h") -> (s? t:f=w924:T1)
                    n212 = local write "part"(w924) -> ()
                    "Step 2H" <- TRUE
                  }
                  frame "i" {
                    n213 = Multiply(x=0, y=w940) -> (x*y=w941:dbl)
                    n214 = for {
                      N: 1 -> [_]
                      n215 = local read "Pulses M1"() -> (w946:dbl)
                      n216 = local read "Pulses M2"() -> (w945:dbl)
                      n217 = local write "Has encoders been reset?"(enum16{"don't reset", "reset"}."reset") -> ()
                      n218 = Equal To 0?(x=w945) -> (x = 0?=w951:bool)
                      n219 = Equal To 0?(x=w946) -> (x = 0?=w952:bool)
                      n220 = And(x=w952, y=w951) -> (x .and. y?=w950:bool)
                      n221 = Select(t=T1."j", s=w950, f=T1."i") -> (s? t:f=w944:T1)
                      n222 = local write "part"(w944) -> ()
                    }
                    n223 = Multiply(x=0, y=w937) -> (x*y=w938:dbl)
                  }
                  frame "j" {
                    (unwired) 1
                    n224 = Multiply(x=-1, y=w963) -> (x*y=w962:dbl)
                    n225 = local read "length"() -> (w956:dbl)
                    n226 = local read "calc distanc x"() -> (w958:dbl)
                    n227 = Multiply(x=w956, y=10) -> (x*y=w953:dbl)
                    n228 = local write "Has encoders been reset?"(enum16{"don't reset", "reset"}."don't reset") -> ()
                    n229 = local write "x distance currently being travelled"(w956) -> ()
                    n230 = Greater?(x=w958, y=w953) -> (0:w967:bool)
                    n231 = local write "y distance currently being travelled"(0) -> ()
                    n232 = Select(t=T1."nothing", s=w967, f=T1."j") -> (s? t:f=w957:T1)
                    n233 = Multiply(x=-1.08, y=w961) -> (x*y=w960:dbl)
                    n234 = local write "part"(w957) -> ()
                    "Step 2J" <- TRUE
                  }
                  frame "nothing" {
                    n235 = Multiply(x=0, y=w974) -> (x*y=w973:dbl)
                    n236 = Multiply(x=0, y=w972) -> (x*y=w970:dbl)
                  }
                }
              }
              frame True {
                n237 = case shown="\"d\"" "part circle" {
                  frame "a" {
                    n238 = for {
                      N: 1 -> [_]
                      n239 = local read "Pulses M1"() -> (w984:dbl)
                      n240 = local read "Pulses M2"() -> (w983:dbl)
                      n241 = Equal To 0?(x=w984) -> (x = 0?=w987:bool)
                      n242 = Equal To 0?(x=w983) -> (x = 0?=w988:bool)
                      n243 = And(x=w987, y=w988) -> (x .and. y?=w989:bool)
                      n244 = local write "Has encoders been reset?"(enum16{"don't reset", "reset"}."reset") -> ()
                      n245 = Select(t=enum16{"d", "c", "b", "a"}."b", s=w989, f=enum16{"d", "c", "b", "a"}."a") -> (s? t:f=w981:enum16{"d", "c", "b", "a"})
                      n246 = local write "part circle"(w981) -> ()
                      "circle reset" <- TRUE
                    }
                  }
                  frame "b" {
                    n247 = while {
                      stop <- w1000 stop-if-true
                      n248 = local read "x distance currently being travelled"() -> (w995:dbl)
                      n249 = local read "Raduis"() -> (w994:dbl)
                      n250 = local read "Pulses M2"() -> (w991:dbl)
                      n251 = Equal?(x=0, y=w991) -> (x = y?=w990:bool)
                      n252 = local read "Raduis"() -> (w1002:dbl)
                      n253 = Equal?(x=w995, y=w994) -> (x = y?=w993:bool)
                      n254 = local write "x distance currently being travelled"(w1002) -> ()
                      n255 = local read "x distance currently being travelled"() -> (w1001:dbl)
                      n256 = And(x=w993, y=w990) -> (x .and. y?=w999:bool)
                      n257 = Equal?(x=w1001, y=w1002) -> (x = y?=w1000:bool)
                      n258 = Select(t=enum16{"d", "c", "b", "a"}."c", s=w999, f=enum16{"d", "c", "b", "a"}."b") -> (s? t:f=w996:enum16{"d", "c", "b", "a"})
                      n259 = local write "part circle"(w996) -> ()
                    }
                  }
                  frame "c" {
                    n260 = for {
                      N: 1 -> [_]
                      n261 = local read "Pulses M1"() -> (w1007:dbl)
                      n262 = local read "Pulses M2"() -> (w1006:dbl)
                      n263 = Equal To 0?(x=w1007) -> (x = 0?=w1010:bool)
                      n264 = Equal To 0?(x=w1006) -> (x = 0?=w1011:bool)
                      n265 = local write "Has encoders been reset?"(enum16{"don't reset", "reset"}."reset") -> ()
                      n266 = And(x=w1010, y=w1011) -> (x .and. y?=w1012:bool)
                      n267 = Select(t=enum16{"d", "c", "b", "a"}."d", s=w1012, f=enum16{"d", "c", "b", "a"}."c") -> (s? t:f=w1004:enum16{"d", "c", "b", "a"})
                      n268 = local write "part circle"(w1004) -> ()
                    }
                  }
                  frame "d" {
                    n269 = while {
                      i -> [w1014]
                      stop <- w1013 stop-if-true
                      n270 = for {
                        N: 50 -> [_]
                        i -> [w1027]
                        n271 = Increment(x=w1027) -> (x+1=w1026:i32)
                        n272 = Multiply(x=2, y=3.141592653589793) -> (x*y=w1023:dbl)
                        n273 = Divide(x=w1023, y=50) -> (x/y=w1025:dbl)
                        n274 = Multiply(x=w1025, y=w1026) -> (x*y=w1022:dbl)
                        n275 = Cosine(x=w1022) -> (cos(x)=w1021:dbl)
                        n276 = Sine(x=w1022) -> (sin(x)=w1019:dbl)
                        n277 = Multiply(x=w1019, y="Raduis") -> (x*y=w1017:dbl)
                        n278 = Multiply(x=w1021, y="Raduis") -> (x*y=w1018:dbl)
                        n279 = local write "x distance currently being travelled"(w1018) -> ()
                        n280 = local write "y distance currently being travelled"(w1017) -> ()
                      }
                      n281 = Equal?(x=49, y=w1014) -> (x = y?=w1013:bool)
                    }
                  }
                }
              }
            }
            "Numeric" <- 2
          }
        }
      }
    }
    "In drawing mode" <- w124
    n282 = Select(t=w123, s=w101, f=w121) -> (s? t:f=w120:dbl)
    n283 = Select(t=w122, s=w101, f=w119) -> (s? t:f=w118:dbl)
    n284 = And(x=w96, y=w97) -> (x .and. y?=w100:bool)
    n285 = Or(x=w170, y=w100) -> (x .or. y?=w169:bool)
    n286 = Or(x=w169, y="Motor stop") -> (x .or. y?=w171:bool)
    n287 = Or(x=w171, y="stop") -> (x .or. y?=w191:bool)
    n288 = Select(t=0.0, s=w191, f=w118) -> (s? t:f=w188:dbl)
    n289 = call-poly <vilib>:"DAQmx Write.vi"("task/channels in"=w197, "data"=w188, "error in"=w194) -> ("task out"=w198:refnum<k21>, "error out"=w199:errorcluster)  [unwired: 10 in, 1 out]
    n290 = Select(t=0.0 ("s? t:f"), s=w191, f=w120) -> (s? t:f=w189:dbl)
    n291 = call-poly <vilib>:"DAQmx Write.vi"("task/channels in"=w203, "data"=w189, "error in"=w193) -> ("task out"=w202:refnum<k21>, "error out"=w201:errorcluster)  [unwired: 10 in, 1 out]
    n292 = call <vilib>:"DAQmx Wait Until Done.vi"("task/channels in"=w202, "error in"=w201) -> ("error out"=w200:errorcluster)  [unwired: 12 in, 1 out]
    n293 = call <vilib>:"DAQmx Wait Until Done.vi"("task/channels in"=w198, "error in"=w199) -> ("error out"=w196:errorcluster)  [unwired: 12 in, 1 out]
    n294 = case shown="True" w66 {
      tunnel: w67 -> [w205 w206]
      frame False {
        n295 = call-poly <vilib>:"DAQmx Read.vi"("task/channels in"=w205) -> ("data"=w204:dbl)  [unwired: 12 in, 2 out]
        n296 = local write "Pulses M2"(w204) -> ()
      }
      frame True {
        n297 = local read "Has encoders been reset?"() -> (w207:enum16{"don't reset", "reset"})
        n298 = case shown="\"reset\"" w207 {
          tunnel: w206 -> [w209 w213]
          frame "don't reset", Default {
            n299 = call-poly <vilib>:"DAQmx Read.vi"("task/channels in"=w209) -> ("data"=→"Pulses M2":dbl)  [unwired: 12 in, 2 out]
          }
          frame "reset" {
            n300 = call <vilib>:"DAQmx Stop Task.vi"("task/channels in"=w213) -> ("task out"=w212:refnum<k21>)  [unwired: 13 in, 1 out]
            n301 = call <vilib>:"DAQmx Start Task.vi"("task/channels in"=w212) -> ("task out"=w214:refnum<k21>)  [unwired: 13 in, 1 out]
            n302 = call-poly <vilib>:"DAQmx Read.vi"("task/channels in"=w214) -> ("data"=w211:dbl)  [unwired: 12 in, 2 out]
            n303 = local write "Pulses M2"(w211) -> ()
            "Boolean 2" <- TRUE
          }
        }
      }
    }
    n304 = call "Number To Enum.vim"("number"=w114, "enum type"=enum16{"corner", "1st switch", "reverse"}."corner") -> ("number as enum"=→"Shape drawing steps":enum16{"corner", "1st switch", "reverse"})
    n305 = case shown="True" w66 {
      tunnel: w71 -> [w217 w222]
      tunnel: w70 -> [w218 w221]
      tunnel: [w215 w220] -> w69
      frame False {
        n306 = call-poly <vilib>:"DAQmx Read.vi"("task/channels in"=w217, "error in"=w218) -> ("data"=w216:dbl, "error out"=w215:errorcluster)  [unwired: 11 in, 1 out]
        n307 = local write "Pulses M1"(w216) -> ()
      }
      frame True {
        n308 = case shown="\"reset\"" "Has encoders been reset?" {
          tunnel: w222 -> [w226 w233]
          tunnel: w221 -> [w225 w232]
          tunnel: [w223 w234] -> w220
          frame "don't reset", Default {
            n309 = call-poly <vilib>:"DAQmx Read.vi"("task/channels in"=w226, "error in"=w225) -> ("data"=→"Pulses M1":dbl, "error out"=w223:errorcluster)  [unwired: 11 in, 1 out]
          }
          frame "reset" {
            n310 = call <vilib>:"DAQmx Stop Task.vi"("task/channels in"=w233, "error in"=w232) -> ("task out"=w231:refnum<k21>, "error out"=w230:errorcluster)  [unwired: 12 in]
            n311 = call <vilib>:"DAQmx Start Task.vi"("task/channels in"=w231, "error in"=w230) -> ("task out"=w229:refnum<k21>, "error out"=w228:errorcluster)  [unwired: 12 in]
            n312 = call-poly <vilib>:"DAQmx Read.vi"("task/channels in"=w229, "error in"=w228) -> ("data"=w227:dbl, "error out"=w234:errorcluster)  [unwired: 11 in, 1 out]
            n313 = local write "Pulses M1"(w227) -> ()
          }
        }
      }
    }
  }
  n314 = invoke on="motor 1" class="Slide (strict)" method="Reinit To Default"() -> ()  [unwired: 3 in, 3 out]
  n315 = call <vilib>:"Simple Error Handler.vi"("error source (\" \")"="you messed up" ("error source (\" \")"), "error in (no error)"=w48) -> ()  [unwired: 3 in, 5 out]
  n316 = call <vilib>:"Simple Error Handler.vi"("error source (\" \")"="you messed up" ("error source (\" \")"), "error in (no error)"=w45) -> ()  [unwired: 3 in, 5 out]
  n317 = call <vilib>:"DAQmx Clear Task.vi"("task in"=w27, "error in"=w25) -> ()  [unwired: 13 in, 1 out]
  n318 = call <vilib>:"DAQmx Clear Task.vi"("task in"=w17, "error in"=w14) -> ()  [unwired: 13 in, 1 out]
  n319 = call <vilib>:"DAQmx Clear Task.vi"("task in"=w18, "error in"=w15) -> ("error out"=w12:errorcluster)  [unwired: 13 in]
  n320 = call <vilib>:"DAQmx Clear Task.vi"("task in"=w16, "error in"=w13) -> ()  [unwired: 13 in, 1 out]
  n321 = call <vilib>:"Simple Error Handler.vi"("error in (no error)"=w12) -> ()  [unwired: 4 in, 5 out]
  n322 = call <vilib>:"Simple Error Handler.vi"("error source (\" \")"="you messed up" ("error source (\" \")"), "error in (no error)"=w10) -> ()  [unwired: 3 in, 5 out]
